vi "HW_Stream_raw_data_enq_2.vi"(8 "error in":errorcluster, 9 "Queue in":refnum<queue>, 10 "Data flow controls in":T1, 11 "VISA resource name in":refnum<visa-resource-name>) -> (0 "error out":errorcluster, 2 "Data flow controls out":T1, 3 "VISA resource name out":refnum<visa-resource-name>, 4 "Queue out":refnum<queue>)   [LabVIEW 2018, in "Tracker.lvlib"]
uses:
  Tracker.lvlib
  <vilib>/Instr/_visa.llb/VISA Flush IO Buffer Mask.ctl
panel:
  out "VISA resource name out 2":refnum<visa-resource-name>
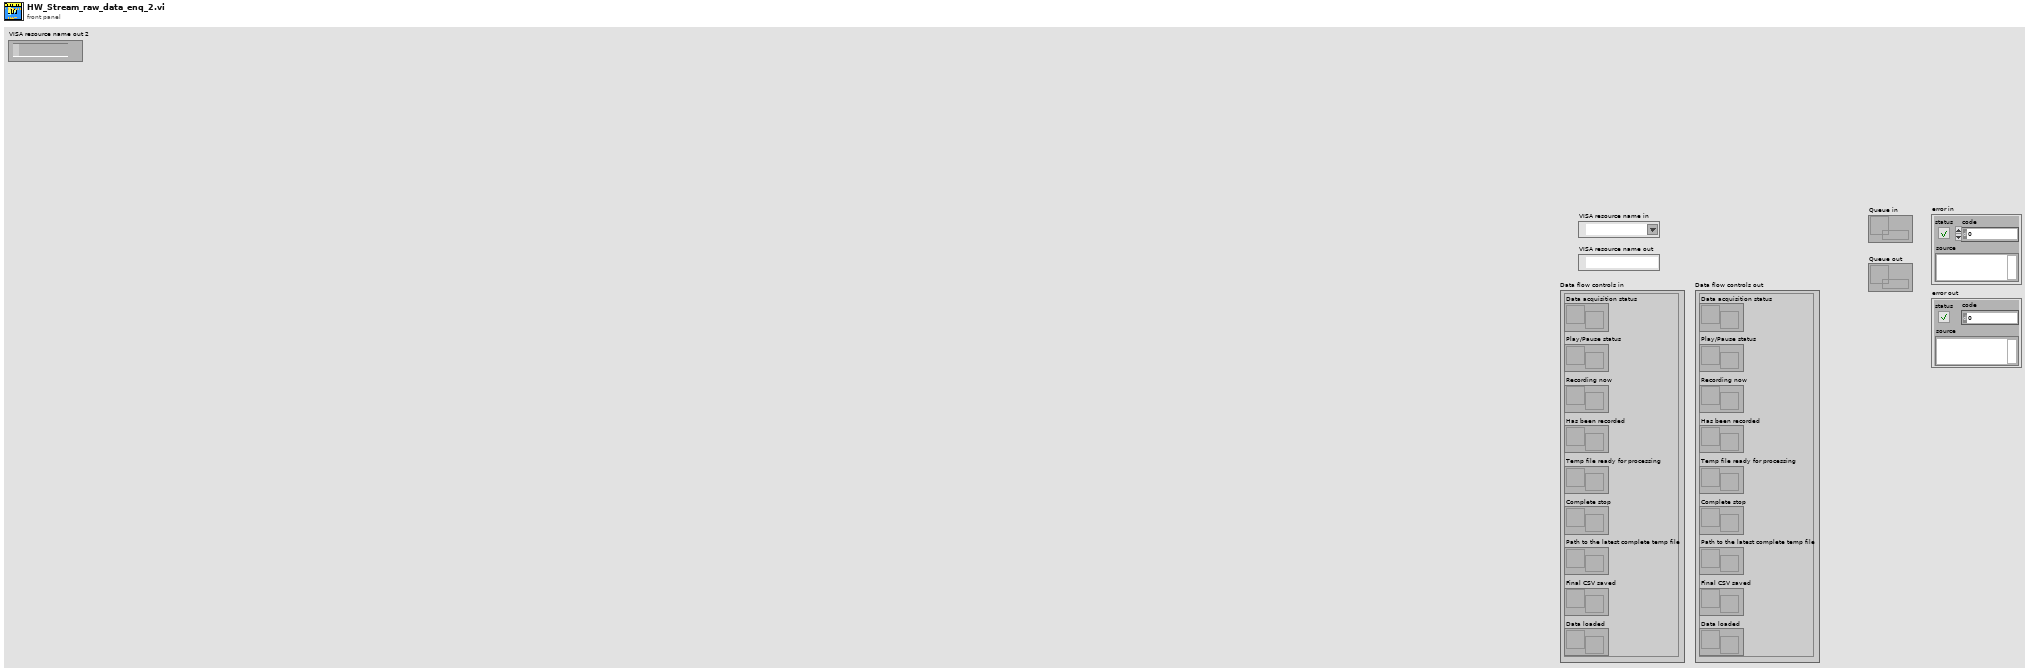
[diagram p1: front panel]
types:
  T1 = cluster{"Data acquisition status":refnum<notifier>, "Play/Pause status":refnum<notifier>, "Complete stop":refnum<notifier>, "Temp file ready for processing":refnum<notifier>, "Has been recorded":refnum<notifier>, "Recording now":refnum<notifier>, "Path to the latest complete temp file":refnum<notifier>, "Final CSV saved":refnum<notifier>, "Data loaded":refnum<notifier>}
  T2 = typedef "VISA Flush IO Buffer Mask.ctl" = u16
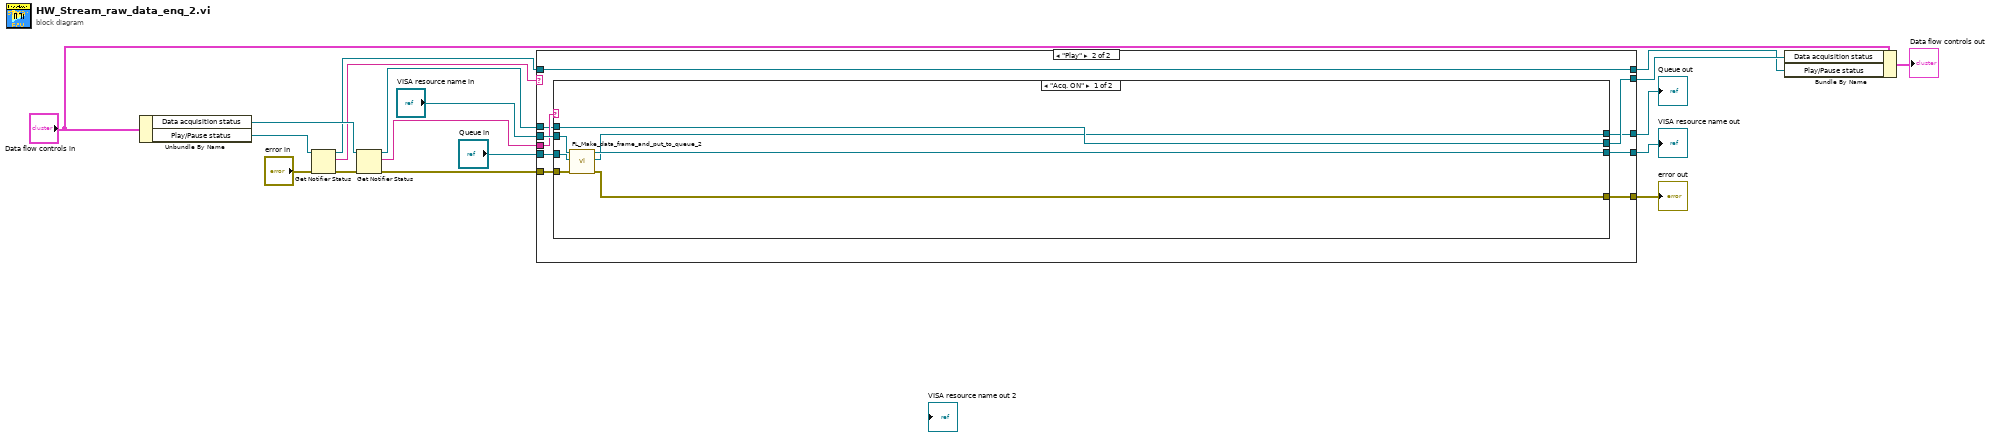
[diagram p0: block diagram]
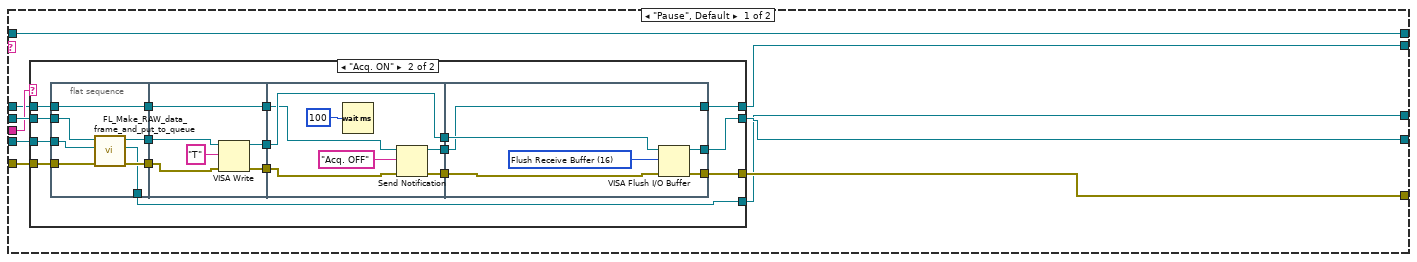
[diagram p2: hidden frame]
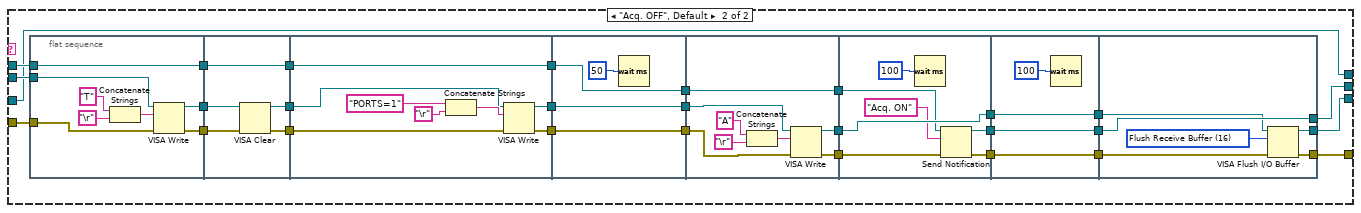
[diagram p4: hidden frame]
diagram:
  n1 = Unbundle By Name("Data flow controls in") -> ("Data acquisition status"=w16:refnum<notifier>, "Play/Pause status"=w15:refnum<notifier>)
  n2 = Get Notifier Status(notifier=w15, error in (no error)="error in") -> (notifier out=w10:refnum<notifier>, current notification=w14:string, error out=w11:errorcluster)  [unwired: 2 out]
  n3 = Get Notifier Status(notifier=w16, error in (no error)=w11) -> (notifier out=w9:refnum<notifier>, current notification=w13:string, error out=w4:errorcluster)  [unwired: 2 out]
  n4 = case shown="\"Play\"" w14 {
    tunnel: [w23 w80] -> w17
    tunnel: "VISA resource name in" -> [w28 w85]
    tunnel: w13 -> [w27 w83]
    tunnel: w10 -> [w25 w81]
    tunnel: w9 -> [w26 w82]
    tunnel: [w22 w79] -> w7
    tunnel: [w25 w81] -> w6
    tunnel: w4 -> [w24 w84]
    tunnel: [w21 w78] -> w3
    tunnel: "Queue in" -> [w19 w77]
    tunnel: [w20 w76] -> w1
    frame "Pause", Default {
      n5 = case shown="\"Acq. ON\"" w27 {
        tunnel: w28 -> [w32 w47]
        tunnel: [w32 w46] -> w23
        tunnel: w26 -> [w31 w40]
        tunnel: [w31 w39] -> w22
        tunnel: w24 -> [w30 w43]
        tunnel: [w30 w42] -> w21
        tunnel: w19 -> [w29 w34]
        tunnel: [w29 w33] -> w20
        frame "Acq. OFF", Default {
        }
        frame "Acq. ON" {
          n6 = flat-sequence {
            tunnel: w40 -> [w56]
            tunnel: w43 -> [w55]
            tunnel: w47 -> [w53]
            tunnel: [w52] -> w37
            tunnel: [w54] -> w36
            tunnel: [w56] -> w35
            tunnel: w34 -> [w51]
            tunnel: [w50] -> w33
            tunnel: [w61] -> w49
            tunnel: [w60] -> w48
            tunnel: [w58] -> w41
            tunnel: w37 -> [w62]
            tunnel: w36 -> [w59]
            tunnel: w35 -> [w58]
            tunnel: w49 -> [w68]
            tunnel: w48 -> [w67]
            tunnel: [w68] -> w45
            tunnel: [w66] -> w44
            tunnel: w41 -> [w64]
            tunnel: [w63] -> w38
            tunnel: [w73] -> w46
            tunnel: w45 -> [w74]
            tunnel: w44 -> [w75]
            tunnel: [w71] -> w42
            tunnel: [w70] -> w39
            tunnel: w38 -> [w70]
            frame #0 {
              n7 = call "FL_Make_RAW_data_frame_and_put_to_queue.vi"("error in"=w55, "Queue in"=w51, "VISA resource name in"=w53) -> ("error out"=w54:errorcluster, "Queue out"=w50:refnum<queue>, "VISA resource name out"=w52:refnum<visa-resource-name>)  [unwired: 6 in]
            }
            frame #1 {
              n8 = VISA Write(VISA resource name=w62, write buffer="T", error in (no error)=w59) -> (VISA resource name out=w61:refnum<visa-resource-name>, error out=w60:errorcluster)  [unwired: 1 out]
            }
            frame #2 {
              n9 = Wait (ms)(milliseconds to wait=u32 100) -> ()  [unwired: 1 out]
              n10 = Send Notification(notification="Acq. OFF", notifier=w64, error in (no error)=w67) -> (notifier out=w63:refnum<notifier>, error out=w66:errorcluster)
            }
            frame #3 {
              w72 = T2 16 items=["Flush Receive Buffer"=16, "Write Transmit Buffer to Device"=32, "Flush Receive Buffer (No I/O)"=64, "Flush Transmit Buffer"=128] ("Mask")
              n11 = VISA Flush I/O Buffer(VISA resource name=w74, mask (16)=w72, error in (no error)=w75) -> (VISA resource name out=w73:refnum<visa-resource-name>, error out=w71:errorcluster)
            }
          }
        }
      }
    }
    frame "Play" {
      n12 = case shown="\"Acq. ON\"" w83 {
        tunnel: w85 -> [w92 w118]
        tunnel: [w91 w117] -> w80
        tunnel: [w89 w116] -> w78
        tunnel: w84 -> [w86 w109]
        tunnel: w82 -> [w90 w104]
        tunnel: [w90 w103] -> w79
        tunnel: w77 -> [w88 w102]
        tunnel: [w87 w102] -> w76
        frame "Acq. ON" {
          n13 = call "FL_Make_data_frame_and_put_to_queue_2.vi"("error in"=w86, "Queue in"=w88, "VISA resource name in"=w92) -> ("error out"=w89:errorcluster, "Queue out"=w87:refnum<queue>, "VISA resource name out"=w91:refnum<visa-resource-name>)  [unwired: 5 in, 1 out]
        }
        frame "Acq. OFF", Default {
          n14 = flat-sequence {
            tunnel: w118 -> [w127]
            tunnel: [w128] -> w115
            tunnel: [w126] -> w114
            tunnel: w109 -> [w122]
            tunnel: [w121] -> w105
            tunnel: w104 -> [w121]
            tunnel: [w133] -> w111
            tunnel: [w132] -> w110
            tunnel: w114 -> [w131]
            tunnel: w115 -> [w130]
            tunnel: [w129] -> w106
            tunnel: w105 -> [w129]
            tunnel: w111 -> [w139]
            tunnel: [w138] -> w113
            tunnel: w110 -> [w137]
            tunnel: [w136] -> w112
            tunnel: [w134] -> w107
            tunnel: w106 -> [w134]
            tunnel: [w144] -> w95
            tunnel: [w143] -> w94
            tunnel: [w145] -> w93
            tunnel: w107 -> [w145]
            tunnel: w113 -> [w144]
            tunnel: w112 -> [w143]
            tunnel: [w148] -> w120
            tunnel: [w147] -> w119
            tunnel: w95 -> [w150]
            tunnel: w94 -> [w149]
            tunnel: [w146] -> w108
            tunnel: w93 -> [w146]
            tunnel: w120 -> [w158]
            tunnel: w119 -> [w159]
            tunnel: w108 -> [w156]
            tunnel: [w157] -> w101
            tunnel: [w159] -> w100
            tunnel: [w155] -> w99
            tunnel: w101 -> [w164]
            tunnel: [w164] -> w98
            tunnel: w100 -> [w163]
            tunnel: [w163] -> w97
            tunnel: w99 -> [w162]
            tunnel: [w162] -> w96
            tunnel: [w166] -> w103
            tunnel: [w170] -> w117
            tunnel: [w169] -> w116
            tunnel: w96 -> [w166]
            tunnel: w97 -> [w165]
            tunnel: w98 -> [w167]
            frame #0 {
              n15 = Concatenate Strings("T" ("write buffer"), "\r") -> (w123:string)
              n16 = VISA Write(VISA resource name=w127, write buffer=w123, error in (no error)=w122) -> (VISA resource name out=w128:refnum<visa-resource-name>, error out=w126:errorcluster)  [unwired: 1 out]
            }
            frame #1 {
              n17 = VISA Clear(VISA resource name=w130, error in (no error)=w131) -> (VISA resource name out=w133:refnum<visa-resource-name>, error out=w132:errorcluster)
            }
            frame #2 {
              n18 = Concatenate Strings("PORTS=1" ("write buffer"), "\r") -> (w140:string)
              n19 = VISA Write(VISA resource name=w139, write buffer=w140, error in (no error)=w137) -> (VISA resource name out=w138:refnum<visa-resource-name>, error out=w136:errorcluster)  [unwired: 1 out]
            }
            frame #3 {
              n20 = Wait (ms)(milliseconds to wait=u32 50) -> ()  [unwired: 1 out]
            }
            frame #4 {
              n21 = Concatenate Strings("A" ("write buffer"), "\r") -> (w151:string)
              n22 = VISA Write(VISA resource name=w150, write buffer=w151, error in (no error)=w149) -> (VISA resource name out=w147:refnum<visa-resource-name>, error out=w148:errorcluster)  [unwired: 1 out]
            }
            frame #5 {
              n23 = Wait (ms)(milliseconds to wait=u32 100) -> ()  [unwired: 1 out]
              n24 = Send Notification(notification="Acq. ON", notifier=w156, error in (no error)=w158) -> (notifier out=w155:refnum<notifier>, error out=w157:errorcluster)
            }
            frame #6 {
              n25 = Wait (ms)(milliseconds to wait=u32 100) -> ()  [unwired: 1 out]
            }
            frame #7 {
              w168 = T2 16 items=["Flush Receive Buffer"=16, "Write Transmit Buffer to Device"=32, "Flush Receive Buffer (No I/O)"=64, "Flush Transmit Buffer"=128] ("Mask")
              n26 = VISA Flush I/O Buffer(VISA resource name=w165, mask (16)=w168, error in (no error)=w167) -> (VISA resource name out=w170:refnum<visa-resource-name>, error out=w169:errorcluster)
            }
          }
        }
      }
    }
  }
  "VISA resource name out" <- w17
  "error out" <- w3
  "Queue out" <- w1
  n27 = Bundle By Name(cluster="Data flow controls in", "Data acquisition status"=w7, "Play/Pause status"=w6) -> (→"Data flow controls out":T1)
